vi "PPL_ActionVIOnRecompile_InlineAsync.vi"(8 "error in":errorcluster, 9 "Timeout (ms)":u32, 10 "Runtime Configurable Section Path":string, 11 "Device Item Ref in":T1 format="%.0x") -> (0 "error out":errorcluster)   [LabVIEW 2020]
uses:
  <vilib>/NI VeriStand/Custom Device API/Custom Device Item Ref.ctl
  <vilib>/NI VeriStand/Custom Device API/Block Data Reference.ctl
  <vilib>/NI VeriStand/Custom Device API/Data Reference.ctl
  <vilib>/NI VeriStand/Custom Device API/Custom Device Channel Type.ctl
  <vilib>/NI VeriStand/Custom Device API/Get Item Property (Variant).vi
  <vilib>/NI VeriStand/Execution/CustomDevice/NI VeriStand - Send Custom Device Message (Byte Array).vi
  <vilib>/NI VeriStand/Custom Device API/Custom Device API.lvlib
  <vilib>/NI/NIVS Inline Async API/_Data Access System Explorer/Data Access System Explorer.lvlib
  <vilib>/NI VeriStand/Execution/CustomDevice/NI_VS Custom Device ExecutionAPI.lvlib
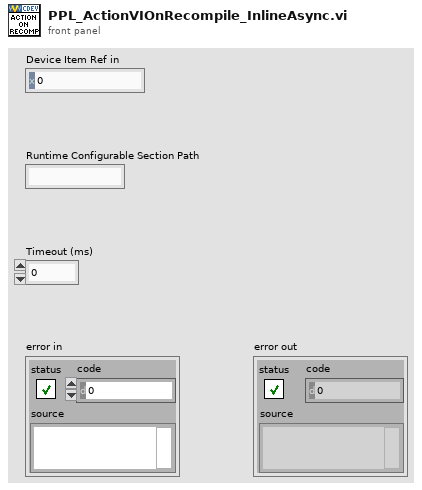
[diagram p1: front panel]
types:
  T1 = typedef "Custom Device API.lvlib/Custom Device Item Ref.ctl" = u64
  T2 = typedef "Custom Device API.lvlib/Custom Device Channel Type.ctl" = enum16{"Input", "Output"}
  T3 = cluster{"Name":string, "Type":enum16{"Output/Write", "Input/Read", "Input/ReadWrite"}, "VS Refs":T1[]}
  T4 = enum16{"Output/Write", "Input/Read", "Input/ReadWrite"}
  T5 = typedef "Custom Device API.lvlib/Block Data Reference.ctl" = cluster{"Data Reference":T6, "Offset":u64, "Length":u64}
  T6 = typedef "Custom Device API.lvlib/Data Reference.ctl" = i32
  T7 = cluster{"Read":cluster{"Refs":T5[], "Values":dbl[]}[], "Write":cluster{"Refs":T5[], "Values":dbl[]}[], "ReadWrite":cluster{"Refs":T6[], "Values":dbl[], "Reset Values":dbl[]}[], "LUT":variant}
  T8 = cluster{"Name":string, "Async Init Timeout":u16, "Compiled.InlineAsync.Settings":cluster{"Read":cluster{"Refs":T5[], "Values":dbl[]}[], "Write":cluster{"Refs":T5[], "Values":dbl[]}[], "ReadWrite":cluster{"Refs":T6[], "Values":dbl[], "Reset Values":dbl[]}[], "LUT":variant}}
  T9 = typedef "Custom Device API.lvlib/Custom Device Item Info.ctl" = cluster{"Name":string, "Is Channel":bool, "GUID":string, "Is Waveform":bool}
  T10 = cluster{"Name":string, "Type":enum16{"Output/Write", "Input/Read", "Input/ReadWrite"}, "VS Refs":T1[]}[]
  T11 = typedef "NI_VS Custom Device ExecutionAPI.lvlib/Custom Device Ref.ctl" = refnum<k24>
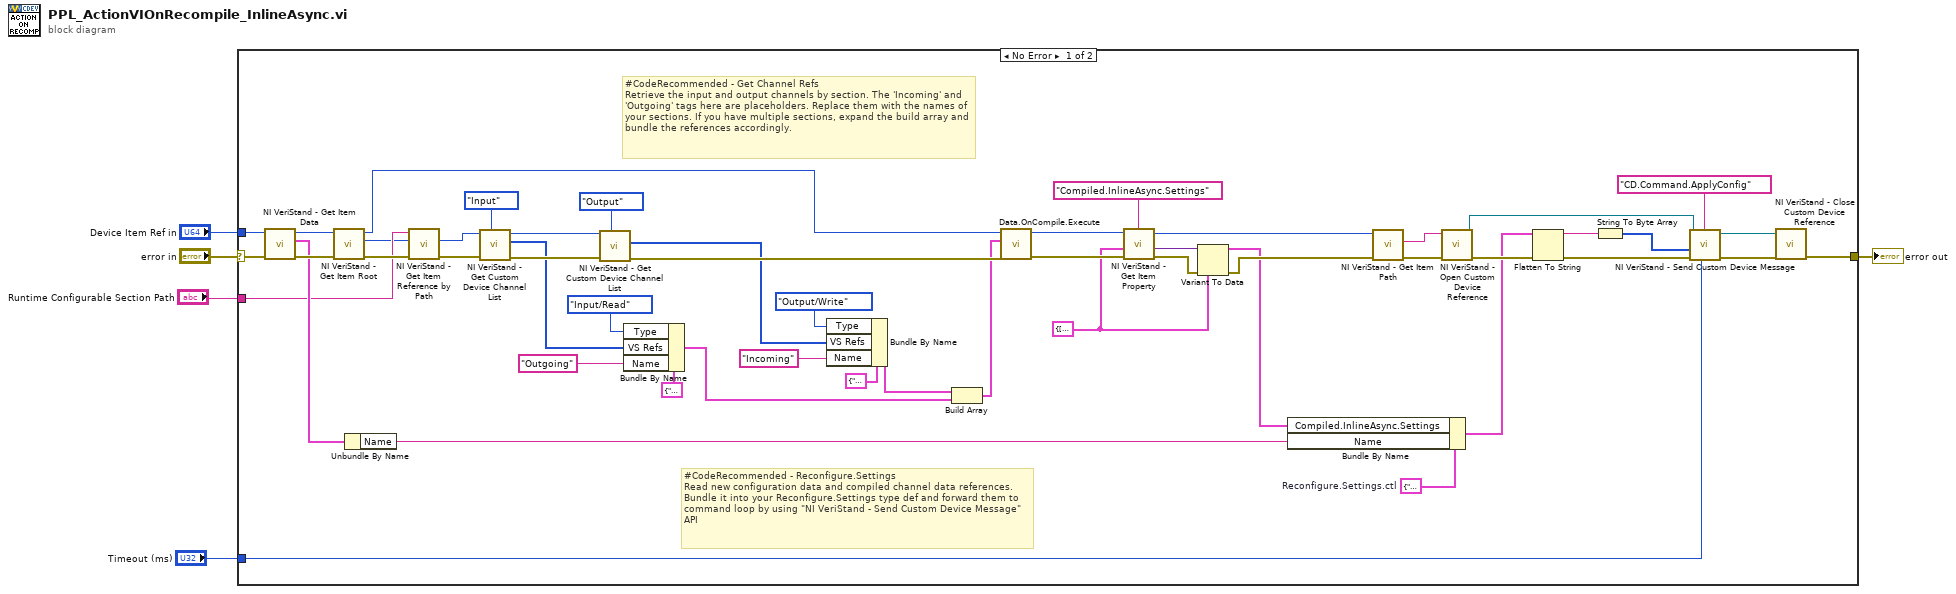
[diagram p0: block diagram]
diagram:
  n1 = case shown="No Error" "error in" {
    selector: "error in" -> [w56 w57]
    tunnel: [w46 w57] -> w4
    tunnel: "Device Item Ref in" -> [w42 _]
    tunnel: "Runtime Configurable Section Path" -> [w30 _]
    tunnel: "Timeout (ms)" -> [w12 _]
    frame No Error {
      w10 = T7 {"Read"=[], "Write"=[], "ReadWrite"=[], "LUT"=variant} ("Compiled.InlineAsync.Settings")
      w23 = T8 {"Name"="", "Async Init Timeout"=0, "Compiled.InlineAsync.Settings"={"Read"=[], "Write"=[], "ReadWrite"=[], "LUT"=variant}}  # Reconfigure.Settings.ctl
      # "#CodeRecommended - Get Channel Refs\nRetrieve the input and output channels by section. The 'Incoming' and 'Outgoing' tags here are placeholders. Replace them with the names of your sections. If you have multiple sections, expand the build array and bundle the references accordingly."
      # "#CodeRecommended - Reconfigure.Settings\nRead new configuration data and compiled channel data references. Bundle it into your Reconfigure.Settings type def and forward them to command loop by using \"NI VeriStand - Send Custom Device Message\" API"
      n2 = call <vilib>:"NI VeriStand - Get Item Data.vi"("error in (no error)"=w56, "Item Ref in"=w42) -> ("error out"=w55:errorcluster, "Item Info"=w41:T9, "Item Ref out"=w7:T1)  [unwired: 6 in, 1 out]
      n3 = call <vilib>:"NI VeriStand - Get Item Root.vi"("error in (no error)"=w55, "Item Ref in"=w7) -> ("error out"=w43:errorcluster, "Root Ref out"=w8:T1, "Item Ref out"=w6:T1)  [unwired: 6 in, 1 out]
      n4 = Unbundle By Name(w41) -> ("Name"=w40:string)
      n5 = call <vilib>:"NI VeriStand - Get Item Reference by Path.vi"("error in (no error)"=w43, "Root Ref"=w8, "Item Path in"=w30) -> ("error out"=w54:errorcluster, "Item Ref"=w29:T1)  [unwired: 5 in, 2 out]
      n6 = call <vilib>:"NI VeriStand - Get Custom Device Channel List.vi"("Channel Type"=Custom_Device_Channel_Type."Input", "error in (no error)"=w54, "Device Ref in"=w29) -> ("error out"=w53:errorcluster, "Specified Channel Ref List"=w25:T1[], "Device Ref out"=w26:T1)  [unwired: 6 in]
      n7 = call <vilib>:"NI VeriStand - Get Custom Device Channel List.vi"("Channel Type"=Custom_Device_Channel_Type."Output", "error in (no error)"=w53, "Device Ref in"=w26) -> ("error out"=w52:errorcluster, "Specified Channel Ref List"=w24:T1[])  [unwired: 6 in, 1 out]
      n8 = Bundle By Name(cluster=T3 {"Name"="", "Type"=enum."Output/Write", "VS Refs"=[]} ("Group"), "Type"=T4."Input/Read", "VS Refs"=w25, "Name"="Outgoing" ("Item Name")) -> (w31:T3)
      n9 = Bundle By Name(cluster=T3 {"Name"="", "Type"=enum."Output/Write", "VS Refs"=[]} ("Group"), "Type"=T4."Output/Write", "VS Refs"=w24, "Name"="Incoming" ("Item Name")) -> (w36:T3)
      n10 = Build Array(w36, w31) -> (w34:T10)
      n11 = call <vilib>:"Data.OnCompile.Execute.vi"("error in"=w52, "VS Ref Groups"=w34, "Custom Device Ref"=w6) -> ("error out"=w49:errorcluster, "Custom Device Ref"=w19:T1)  [unwired: 7 in]
      n12 = call-poly <vilib>:"NI VeriStand - Get Item Property.vi"("error in (no error)"=w49, "Default Value"=w10, "Property Name"="Compiled.InlineAsync.Settings", "Item Ref in"=w19) -> ("error out"=w44:errorcluster, "Value"=w17:variant, "Item Ref out"=w11:T1)  [unwired: 4 in, 1 out]
      n13 = Variant To Data(error in=w44, type=w10, Variant=w17) -> (data=w9:T7, error out=w51:errorcluster)
      n14 = Bundle By Name(cluster=w23, "Compiled.InlineAsync.Settings"=w9, "Name"=w40) -> (w16:T8)
      n15 = call <vilib>:"NI VeriStand - Get Item Path.vi"("error in (no error)"=w51, "Item Ref in"=w11) -> ("error out"=w50:errorcluster, "Path"=w22:string)  [unwired: 6 in, 2 out]
      n16 = call <vilib>:"NI VeriStand - Open Custom Device Reference.vi"("error in (no error)"=w50, "Custom Device Path"=w22) -> ("error out"=w48:errorcluster, "Custom Device"=w21:T11)  [unwired: 8 in]
      n17 = Flatten To String(anything=w16, error in (no error)=w48) -> (data string=w15:string, error out=w47:errorcluster)  [unwired: 2 in, 1 out]
      n18 = String To Byte Array(string=w15) -> (unsigned byte array=w14:u8[])
      n19 = call-poly <vilib>:"NI VeriStand - Send Custom Device Message.vi"("Timeout ms (5000)"=w12, "error in (no error)"=w47, "Data"=w14, "Command"="CD.Command.ApplyConfig", "Custom Device in"=w21) -> ("error out"=w45:errorcluster, "Custom Device out"=w13:T11)  [unwired: 4 in, 1 out]
      n20 = call <vilib>:"NI VeriStand - Close Custom Device Reference.vi"("error in (no error)"=w45, "Custom Device"=w13) -> ("error out"=w46:errorcluster)  [unwired: 9 in]
    }
    frame Error {
    }
  }
  "error out" <- w4
